vi "Get File System Separator.vi"() -> (0 "Path Separator":string)   [LabVIEW 2020]
doc: "Returns the path separator for the current platform.\n(i.e. '/' on Unix , ':' on the Mac, and '\\' on the PC)."
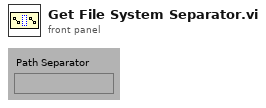
[diagram p1: front panel]
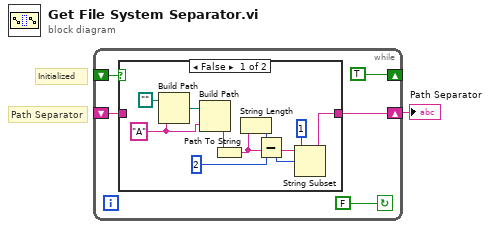
[diagram p0: block diagram]
diagram:
  # "Path Separator"
  # "Initialized"
  n1 = while {
    shift-left: _ -> [w5]
    shift-right: [w4] -> w1
    shift-left: _ -> [w3]
    shift-right: [TRUE] -> _
    stop <- FALSE continue-if-true
    n2 = case shown="False" w3 {
      tunnel: w5 -> [_ w17]
      tunnel: [w7 w17] -> w4
      frame False {
        w14 = "A"
        n3 = Build Path(base path=path "", name or relative path=w14) -> (appended path=w15:path)
        n4 = Build Path(base path=w15, name or relative path=w14) -> (appended path=w13:path)
        n5 = Path To String(path=w13) -> (string=w12:string)
        n6 = String Length(string=w12) -> (length=w11:i32)
        n7 = Subtract(x=w11, y=2) -> (x-y=w10:i32)
        n8 = String Subset(string=w12, offset (0)=w10, length (rest)=1) -> (substring=w7:string)
      }
      frame True {
      }
    }
  }
  "Path Separator" <- w1
